vi "Test Get Class.vi"(8 "error in (no error)":errorcluster, 11 "TestCase in":refnum<class "Test Factory Pattern.lvclass">) -> (0 "error out":errorcluster, 3 "TestCase out":refnum<class "Test Factory Pattern.lvclass">)   [LabVIEW 2020, in "Test Factory Pattern.lvclass"]
uses:
  Test Factory Pattern.lvclass
  26f25a29-ac62-4694-8fa4-7c9b7c9e1776.vi
  <vilib>/Comparison/Equal/Equal Functor/Equal Functor.lvclass
  <vilib>/addons/_JKI Toolkits/VI Tester/TestCase.llb/TestCase.lvclass
  C:/Program Files (x86)/National Instruments/LabVIEW 2020/vi.lib/addons/_JKI Toolkits/VI Tester/TestCase.llb/TestCase.lvclass
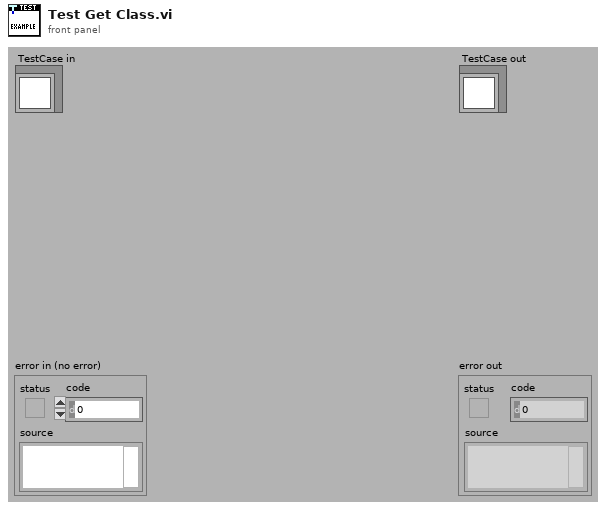
[diagram p1: front panel]
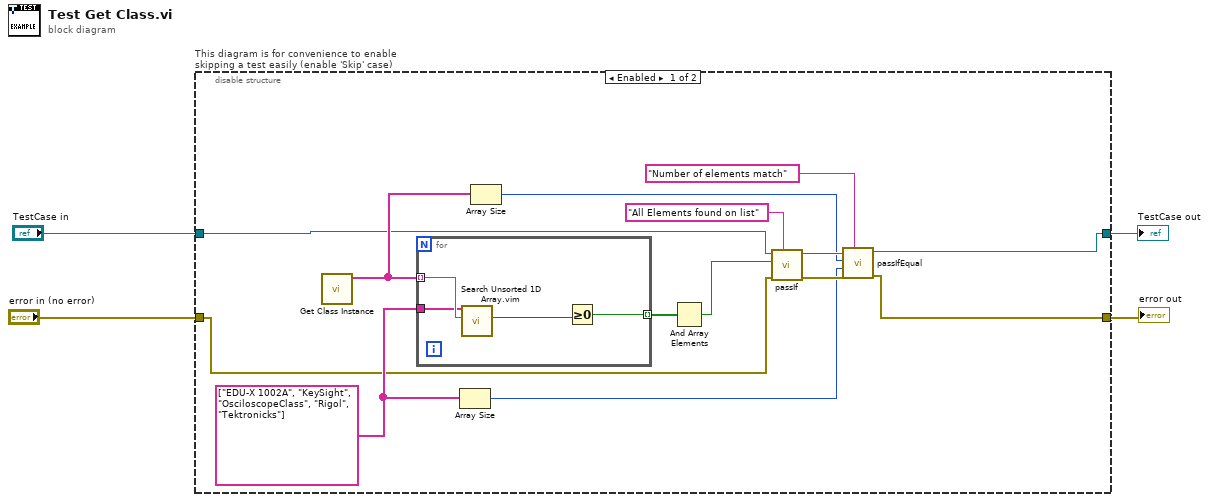
[diagram p0: block diagram]
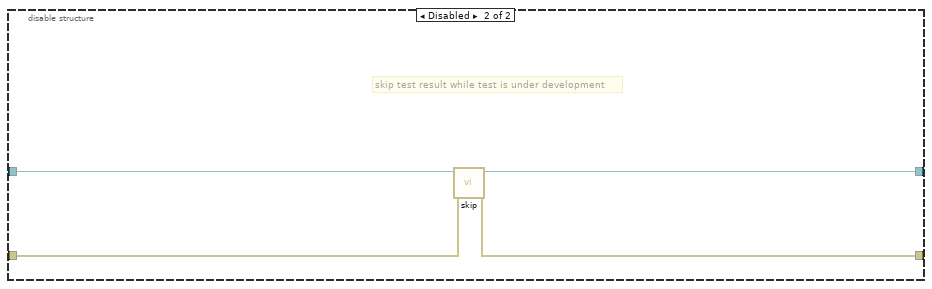
[diagram p2: hidden frame]
diagram:
  n1 = disable-structure "This diagram is for convenience to enable skipping a test easily (enable 'Skip' case)" shown="Enabled" {
    disable-tunnel: "TestCase in" -> [w11 w26]
    disable-tunnel: [w6 w24] -> w1
    disable-tunnel: [w5 w25] -> w3
    disable-tunnel: "error in (no error)" -> [w10 w23]
    frame Enabled {
      w18 = string[] ["EDU-X 1002A", "KeySight", "OsciloscopeClass", "Rigol", "Tektronicks"] ("Classes")
      n2 = call "Get Class Instance.vi"() -> ("Classes"=w16:string[])  [unwired: 11 in]
      n3 = for {
        tunnel: w18 -> [w19]
        tunnel: w16 -> [w20] mode=indexing
        tunnel: [w22] -> w17 mode=indexing
        n4 = call "Search Unsorted 1D Array.vim"("element"=w20, "unsorted 1D array"=w19) -> ("index of element"=w21:i32)  [unwired: 9 in]
        n5 = Greater Or Equal To 0?(x=w21) -> (x >= 0?=w22:bool)
      }
      n6 = Array Size(array=w18) -> (size(s)=w13:i32)
      n7 = Array Size(array=w16) -> (size(s)=w12:i32)
      n8 = And Array Elements(Boolean array=w17) -> (logical AND=w8:bool)
      n9 = call-dynamic "passIf.vi"("custom report message (\"\")"="All Elements found on list" ("custom report message (\"\")"), "error in (no error)"=w10, "pass"=w8, "TestCase in"=w11) -> ("error out"=w14:errorcluster, "TestCase out"=w15:refnum<class "Test Factory Pattern.lvclass">)  [unwired: 6 in]
      n10 = call-dynamic "passIfEqual.vi"("custom report message (\"\")"="Number of elements match" ("custom report message (\"\")"), "error in (no error)"=w14, "y"=w13, "x"=w12, "TestCase in"=w15) -> ("error out"=w5:errorcluster, "TestCase out"=w6:refnum<class "Test Factory Pattern.lvclass">)  [unwired: 5 in]
    }
    frame Disabled {
      # "skip test result while test is under development"
      n11 = call <vilib>:"skip.vi"("error in (no error)"=w23, "TestCase in"=w26) -> ("error out"=w25:errorcluster, "TestCase out"=w24:refnum<class "Test Factory Pattern.lvclass">)  [unwired: 8 in]
    }
  }
  "error out" <- w3
  "TestCase out" <- w1
